vi "MotorPosCtrl(deg)(1).vi"(7 "WorkRange":dbl=100.0 format="%#_13g", 8 "error in (no error)":errorcluster, 10 "Reset Button":bool, 11 "Target(deg)":dbl(knob) scale=90.0..-90.0) -> (0 "error out":errorcluster, 3 "PresentPOS(deg)":dbl(knob) scale=90.0..-90.0, 4 "In Range?":bool)   [LabVIEW 2019, in "MotorPID.lvlib"]
uses:
  MotorPID.lvlib
  KNRm_ReMi_OS5.lvlibp/KNRm_ReMi_Toolkit/IO/LowLevel/IO_Channel_Motor.ctl
  <vilib>/addons/control/pid/pid.llb/PID (DBL).vi
  <vilib>/addons/control/pid/NI_PID_pid.lvlib
  KNRm_ReMi_OS5.lvlibp
panel:
  out "Waveform Chart":cluster{dbl, "Counter Value":i32}(graph)
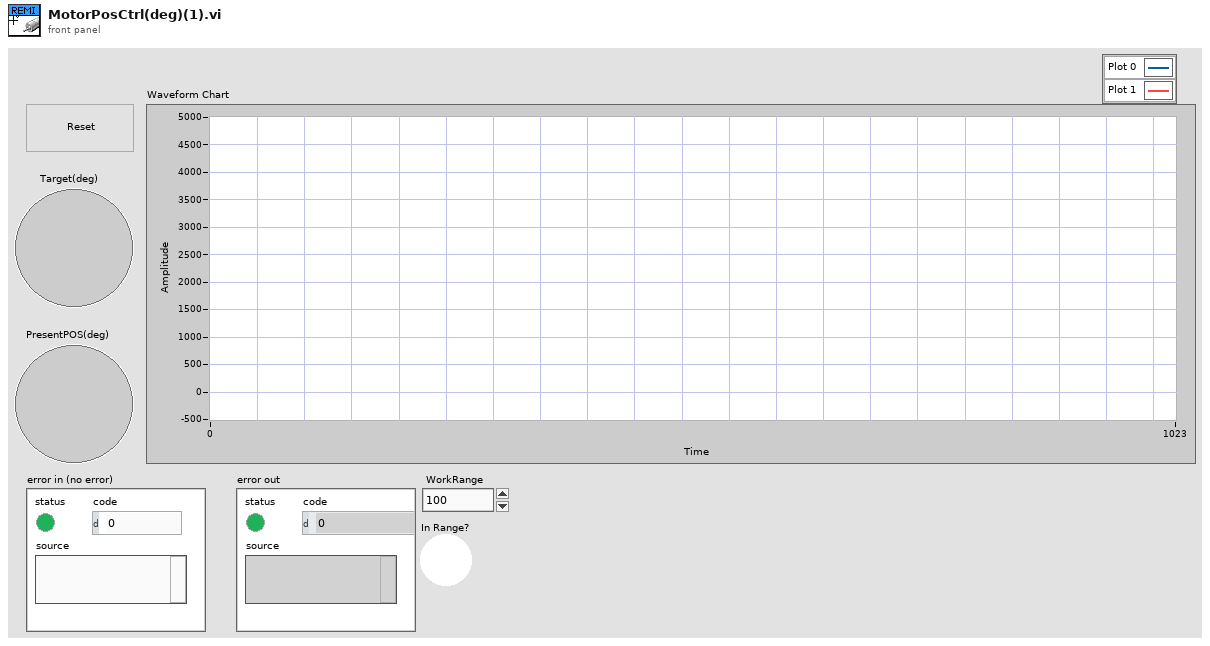
[diagram p1: front panel]
types:
  T1 = cluster{"proportional gain (Kc)":dbl, "integral time (Ti, min)":dbl, "derivative time (Td, min)":dbl}
  T2 = typedef "KNRm_ReMi_OS5.lvlibp/IO_Channel_Motor.ctl" = enum16{"M1", "M2", "M3", "M4"}
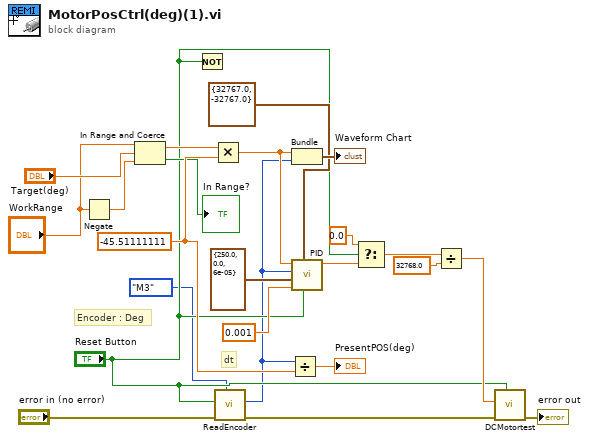
[diagram p0: block diagram]
diagram:
  w15 = -45.51111111 ("y")
  # "dt"
  # "Encoder : Deg"
  n1 = Negate(x="WorkRange") -> (-x=w11:dbl)
  n2 = In Range and Coerce(upper limit="WorkRange", x="Target(deg)", lower limit=w11) -> (coerced(x)=w10:dbl, In Range?=→"In Range?":bool)
  n3 = Not(x="Reset Button") -> ()  [unwired: 1 out]
  n4 = Multiply(x=w10, y=w15) -> (x*y=w22:dbl)
  n5 = call "ReadEncoder.vi"("Channel"=IO_Channel_Motor."M3", "error in"="error in (no error)", "Reset"="Reset Button") -> ("error out"=w1:errorcluster, "ENC (count)"=w2:i32)  [unwired: 7 in]
  n6 = Divide(x=w2, y=w15) -> (x/y=→"PresentPOS(deg)":dbl)
  n7 = Bundle(w22, "ENC (count)"=w2) -> (→"Waveform Chart":cluster{dbl, "ENC (count)":i32})  [unwired: 1 in]
  n8 = call-poly <vilib>:"PID.vi"("reinitialize? (F)"="Reset Button", "output range"=cluster{"output high":dbl, "output low":dbl} {"output high"=32767.0, "output low"=-32767.0}, "dt (s)"=0.001, "PID gains"=T1 {"proportional gain (Kc)"=250.0, "integral time (Ti, min)"=0.0, "derivative time (Td, min)"=6e-05}, "process variable"=w2, "setpoint"=w22) -> ("output"=w20:dbl)  [unwired: 4 in, 1 out]
  n9 = Select(t=0.0, s="Reset Button", f=w20) -> (s? t:f=w6:dbl)
  n10 = Divide(x=w6, y=32768.0 ("output high")) -> (x/y=w7:dbl)
  n11 = call "DCMotortest.vi"("Reset"="Reset Button", "error in"=w1, "PWM"=w7) -> ("error out"=→"error out":errorcluster)  [unwired: 7 in, 1 out]
